vi "Shooter De-Jam.vi"(11 "In Value":dbl) -> (3 "Out Value":dbl)   [LabVIEW 2012]
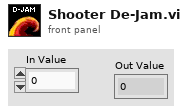
[diagram p1: front panel]
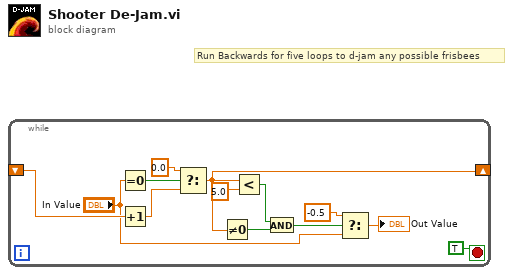
[diagram p0: block diagram]
diagram:
  # "Run Backwards for five loops to d-jam any possible frisbees"
  n1 = while {
    shift-right: [w1] -> _
    shift-left: _ -> [w13]
    stop <- TRUE stop-if-true
    n2 = Equal To 0?(x="In Value") -> (x = 0?=w12:bool)
    n3 = Increment(x=w13) -> (x+1=w10:dbl)
    n4 = Select(t=0.0, s=w12, f=w10) -> (s? t:f=w1:dbl)
    n5 = Not Equal To 0?(x=w1) -> (x != 0?=w5:bool)
    n6 = Less?(x=w1, y=5.0) -> (x < y?=w4:bool)
    n7 = And(x=w4, y=w5) -> (x .and. y?=w3:bool)
    n8 = Select(t=-0.5, s=w3, f="In Value") -> (s? t:f=→"Out Value":dbl)
  }
